vi "Close.vi"(8 "error in (no error)":errorcluster, 11 "VISA resource name":refnum<visa-resource-name>) -> (0 "error out":errorcluster)   [LabVIEW 2020, in "Newport ESP301.lvlib"]
doc: "Performs an instrument error query before terminating the software connection to the instrument."
uses:
  Newport ESP301.lvlib
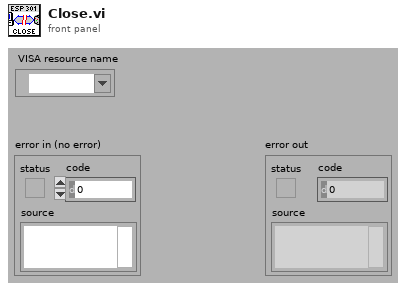
[diagram p1: front panel]
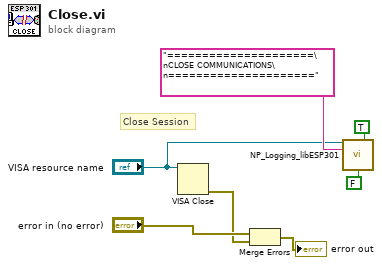
[diagram p0: block diagram]
diagram:
  # "Close Session"
  n1 = VISA Close(VISA resource name="VISA resource name") -> (error out=w6:errorcluster)  [unwired: 1 in]
  n2 = Merge Errors("error in (no error)", w6) -> (→"error out":errorcluster)
  n3 = call "NP_Logging_libESP301.vi"("Instrument Channel"="VISA resource name", "Generic Strings"=TRUE, "String 1 {Write} (in)"="=====================\nCLOSE COMMUNICATIONS\n=====================", "String 2 Enable (T)"=FALSE) -> ()  [unwired: 8 in, 4 out]
